vi "Main.vi"() -> ()   [LabVIEW 2021]
uses:
  <vilib>/Native 3D Graph/xcontrol/3DPC_SurfacePlot.xctl
  State.ctl
  CommCluster.ctl
  CommandCtrl.ctl
  DataCluster.ctl
  ToViewData.ctl
  ToViewCMD.ctl
panel:
  out "3D Graph":refnum<class "Base Datatype.lvclass">[](xcontrol)
  out "length":i32
  out "Stoping":bool
  in  "remote port or service name 2":u16=2137
  in  "address":string="192.168.0.1"
  in  "stop":bool
  in  "Str To Send":string
  out "ReceivedData":string
  in  "Send":bool
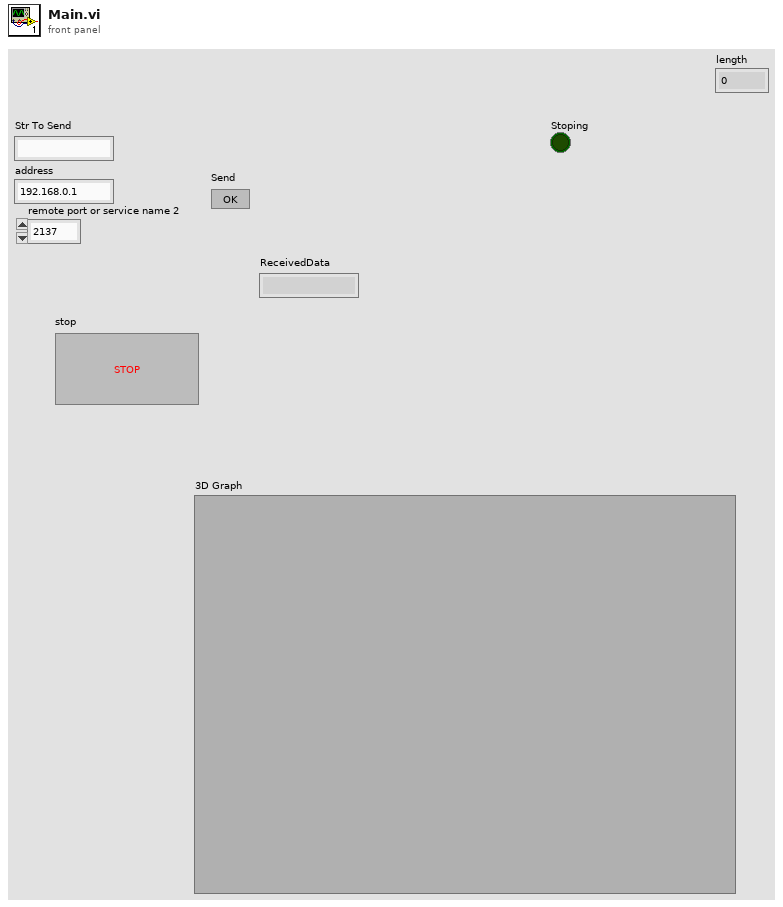
[diagram p1: front panel]
types:
  T1 = typedef "ToViewData.ctl" = cluster{"RecivedStr":string, "Enum":T2}
  T2 = typedef "ToViewCMD.ctl" = enum16{"Exit", "Init", "Update View"}
  T3 = typedef "DataCluster.ctl" = cluster{"connection ID":refnum<k5>, "Str to Send":string, "Received str":string}
  T4 = typedef "CommCluster.ctl" = cluster{"Command":T5, "Data":T3}
  T5 = typedef "CommandCtrl.ctl" = enum16{"Exit", "Init", "Receive TCP", "Send TCP"}
  T6 = typedef "State.ctl" = enum16{"Init", "Idle", "TCP_Read", "TCP_Write", "Exit"}
  T7 = enum16{"Standard", "Buffered", "CRLF", "Immediate"}
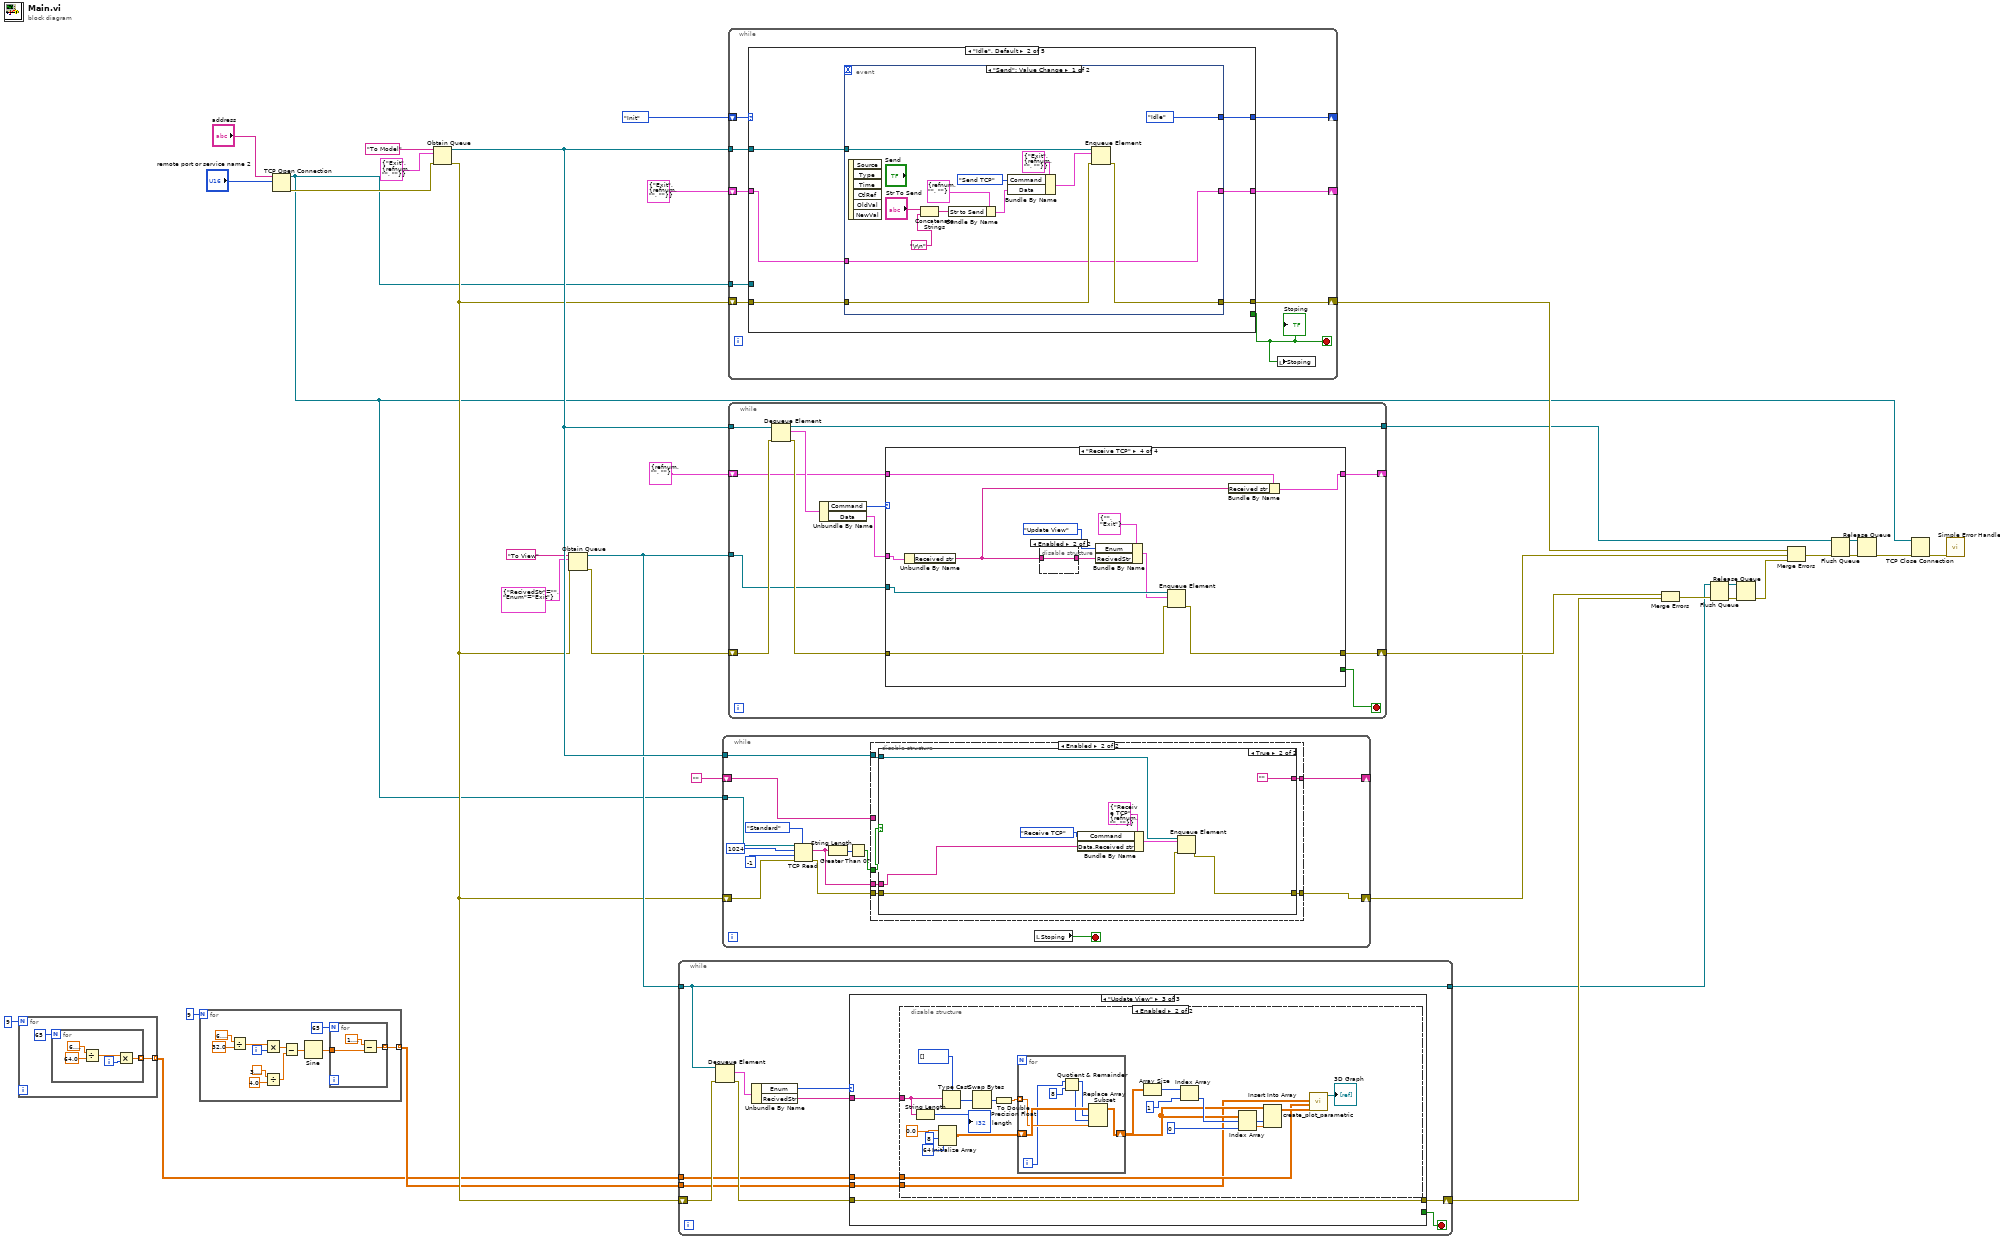
[diagram p0: block diagram]
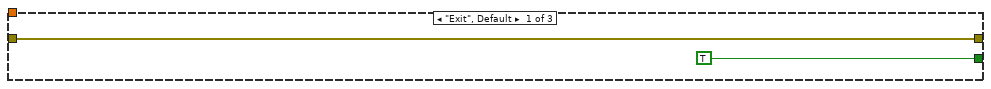
[diagram p2: hidden frame]
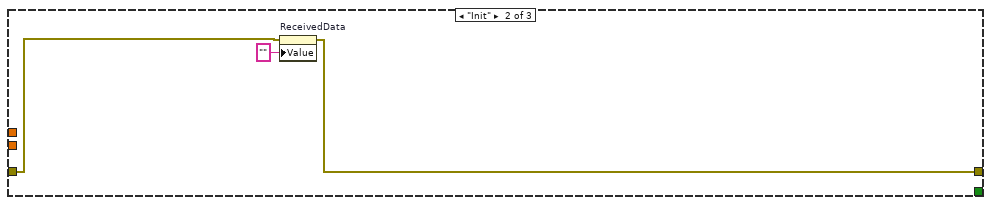
[diagram p3: hidden frame]
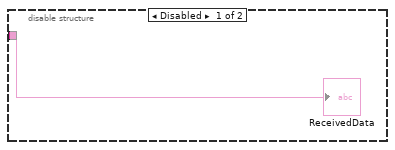
[diagram p4: hidden frame]
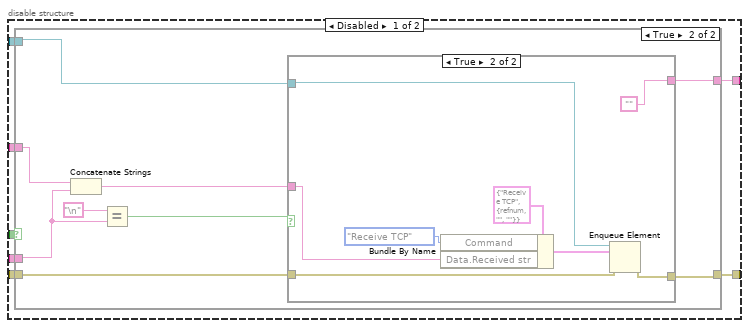
[diagram p5: hidden frame]
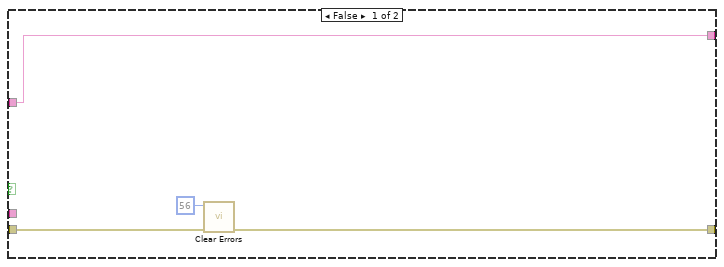
[diagram p6: hidden frame]
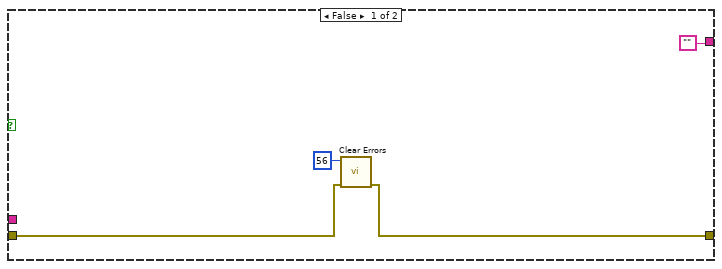
[diagram p8: hidden frame]
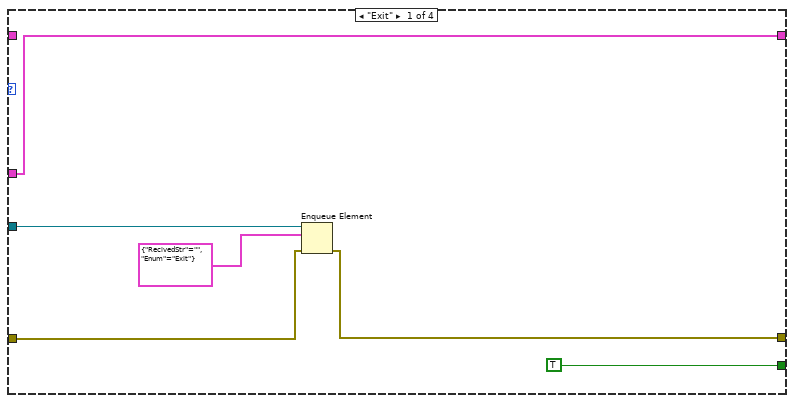
[diagram p9: hidden frame]
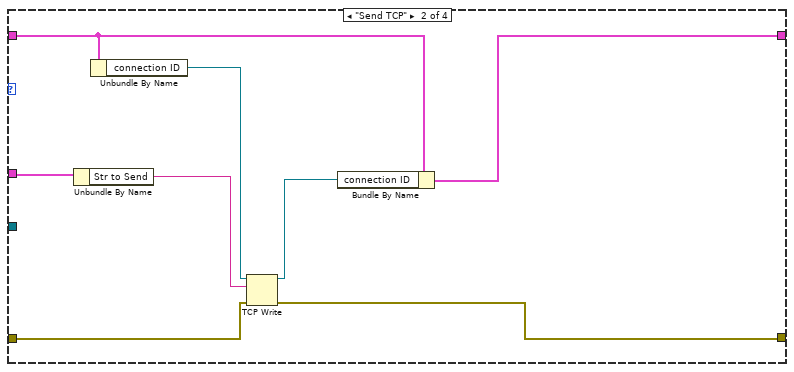
[diagram p10: hidden frame]
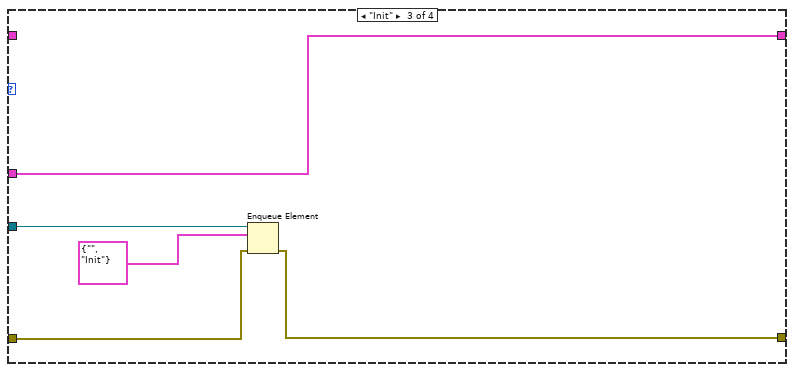
[diagram p11: hidden frame]
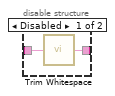
[diagram p12: hidden frame]
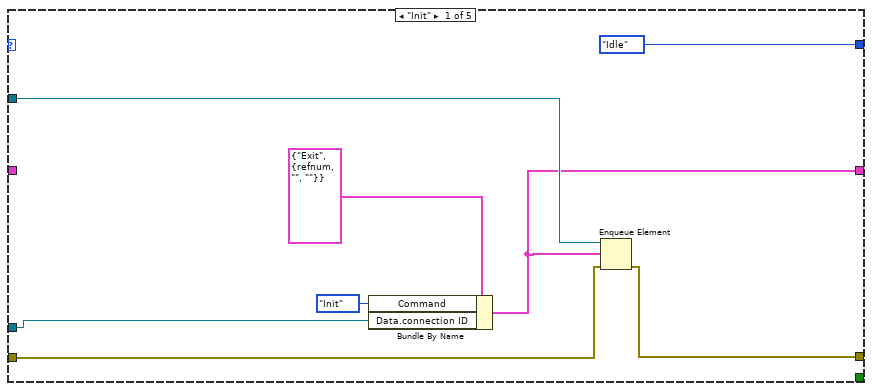
[diagram p13: hidden frame]
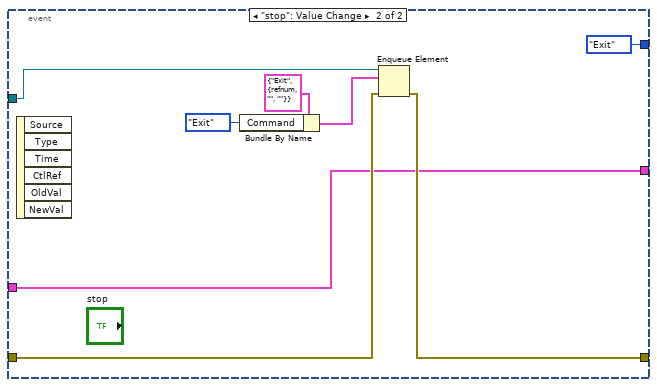
[diagram p14: hidden frame]
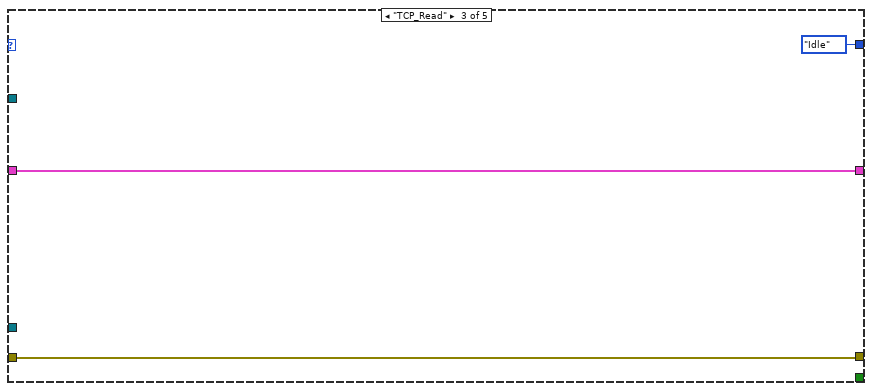
[diagram p15: hidden frame]
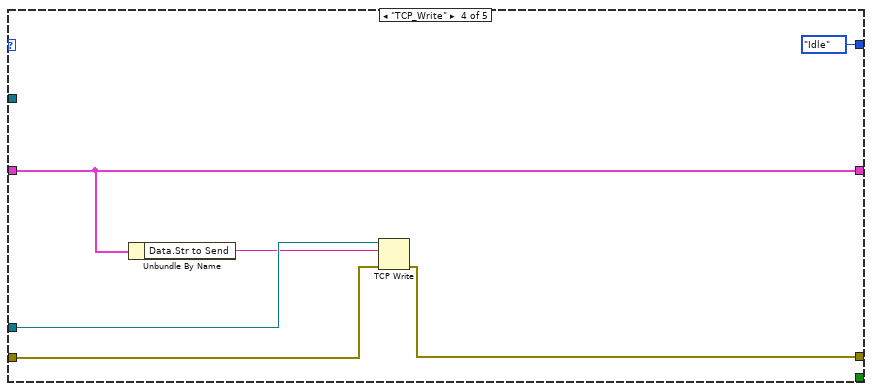
[diagram p16: hidden frame]
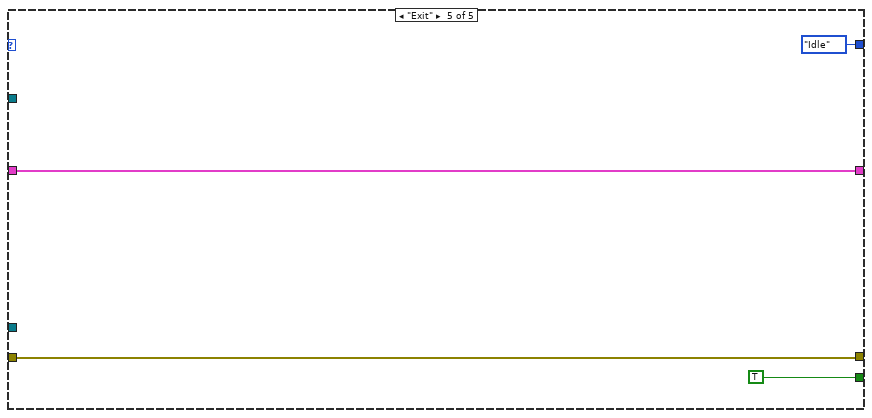
[diagram p17: hidden frame]
diagram:
  n1 = for {
    N: 9 -> [_]
    tunnel: [w36] -> w1 mode=indexing
    n2 = for {
      N: 65 -> [_]
      tunnel: [w39] -> w36 mode=indexing
      i -> [w40]
      n3 = Divide(x=6.283185307179586, y=64.0) -> (x/y=w41:dbl)
      n4 = Multiply(x=w41, y=w40) -> (x*y=w39:dbl)
    }
  }
  n5 = for {
    N: 9 -> [_]
    tunnel: [w44] -> w2 mode=indexing
    i -> [w52]
    n6 = Divide(x=6.283185307179586, y=32.0) -> (x/y=w53:dbl)
    n7 = Multiply(x=w53, y=w52) -> (x*y=w49:dbl)
    n8 = Divide(x=3.141592653589793, y=4.0) -> (x/y=w46:dbl)
    n9 = Subtract(x=w49, y=w46) -> (x-y=w50:dbl)
    n10 = Sine(x=w50) -> (sin(x)=w45:dbl)
    n11 = for {
      N: 65 -> [_]
      tunnel: w45 -> [w56]
      tunnel: [w55] -> w44 mode=indexing
      n12 = Subtract(x=1.5707963267948966, y=w56) -> (x-y=w55:dbl)
    }
  }
  n13 = TCP Open Connection(address="address", remote port or service name="remote port or service name 2") -> (connection ID=w6:refnum<k5>, error out=w28:errorcluster)  [unwired: 3 in]
  n14 = Obtain Queue(name (unnamed)="To Model", element data type=T4 {"Command"=enum."Exit", "Data"={"connection ID"=refnum, "Str to Send"="", "Received str"=""}}, error in (no error)=w28) -> (queue out=w27:refnum<queue>, error out=w22:errorcluster)  [unwired: 2 in, 1 out]
  n15 = Obtain Queue(name (unnamed)="To View", element data type=T1 {"RecivedStr"="", "Enum"=enum."Exit"}, error in (no error)=w22) -> (queue out=w23:refnum<queue>, error out=w25:errorcluster)  [unwired: 2 in, 1 out]
  n16 = while {
    shift-right: [w63] -> w21
    shift-left: w22 -> [w67]
    tunnel: w23 -> [w60]
    tunnel: [w60] -> w18
    tunnel: w2 -> [w59]
    tunnel: w1 -> [w58]
    stop <- w62 stop-if-true
    n17 = Dequeue Element(queue=w60, error in (no error)=w67) -> (element=w66:T1, error out=w64:errorcluster)  [unwired: 1 in, 2 out]
    n18 = Unbundle By Name(w66) -> ("Enum"=w65:T2, "RecivedStr"=w61:string)
    n19 = case shown="\"Update View\"" w65 {
      tunnel: w64 -> [w68 w71 w76]
      tunnel: [w68 w70 w76] -> w63
      tunnel: [TRUE _ _] -> w62
      tunnel: w61 -> [_ _ w75]
      tunnel: w59 -> [_ _ w74]
      tunnel: w58 -> [_ _ w73]
      frame "Exit", Default {
      }
      frame "Init" {
        n20 = property on="ReceivedData" class="Str"(error in=w71, "Value"="" ("ReceivedData")) -> (error out=w70:errorcluster)  [unwired: 1 in, 1 out]
      }
      frame "Update View" {
        n21 = disable-structure shown="Enabled" {
          disable-tunnel: w75 -> [w77 w90]
          disable-tunnel: w74 -> [_ w78]
          disable-tunnel: w73 -> [_ w79]
          frame Disabled {
            "ReceivedData" <- w77
          }
          frame Enabled {
            n22 = String Length(string=w90) -> (length=→"length":i32)
            n23 = Initialize Array(0.0 ("element"), 8 ("dimension size"), 64 ("dimension size")) -> (w91:dbl[][])
            n24 = Type Cast(type=u16[] [], x=w90) -> (*(type *) &x=w96:u16[])
            n25 = Swap Bytes(anything=w96) -> (byte swapped=w88:u16[])
            n26 = To Double Precision Float(number=w88) -> (double precision float=w95:dbl[])
            n27 = for {
              tunnel: w95 -> [w100] mode=indexing
              shift-right: [w102] -> w84
              shift-left: w91 -> [w104]
              i -> [w98]
              n28 = Quotient & Remainder(x=w98, y=8 ("x")) -> (x-y*floor(x/y)=w103:i32, floor(x/y)=w101:i32)
              n29 = Replace Array Subset(array=w104, new element=w100, index (row)=w103, index (col)=w101) -> (w102:dbl[][])
            }
            n30 = Array Size(array=w84) -> (size(s)=w87:i32[])
            n31 = Index Array(array=w87, index=1) -> (element=w85:i32)
            n32 = Index Array(array=w84, index (col)=0 ("disabled index (col)")) -> (element=w82:dbl[])  [unwired: 1 in]
            n33 = Insert Into Array(array=w84, index (col)=w85, new element=w82) -> (w80:dbl[][])  [unwired: 1 in]
            n34 = call <vilib>:"create_plot_parametric.vi"("z matrix"=w80, "y matrix"=w79, "x matrix"=w78) -> ("plots out"=→"3D Graph":refnum<class "Base Datatype.lvclass">[])  [unwired: 2 in, 6 out]
          }
        }
      }
    }
  }
  n35 = while {
    shift-right: [w109] -> w13
    shift-left: w22 -> [w116]
    tunnel: w27 -> [w111]
    tunnel: w6 -> [w117]
    shift-right: [w106] -> _
    shift-left: "" -> [w107]
    stop <- w115 stop-if-true
    n36 = TCP Read(connection ID=w117, bytes to read=1024, error in (no error)=w116, 7:T7."Standard" ("mode (standard)"), 9:-1 ("timeout ms (25000)")) -> (data out=w114:string, error out=w110:errorcluster)  [unwired: 1 out]
    n37 = String Length(string=w114) -> (length=w113:i32)
    n38 = Greater Than 0?(x=w113) -> (x > 0?=w112:bool)
    n39 = disable-structure shown="Enabled" {
      disable-tunnel: w114 -> [w125 w153]
      disable-tunnel: w112 -> [w124 w151]
      disable-tunnel: w111 -> [w123 w154]
      disable-tunnel: w110 -> [w122 w152]
      disable-tunnel: [w121 w150] -> w109
      disable-tunnel: w107 -> [w120 _]
      disable-tunnel: [w119 w149] -> w106
      frame Disabled {
        n40 = case shown="True" w124 {
          tunnel: w125 -> [_ w132]
          tunnel: w123 -> [_ w138]
          tunnel: w122 -> [w129 w137]
          tunnel: [w127 w136] -> w121
          tunnel: w120 -> [w128 w133]
          tunnel: [w128 w130] -> w119
          frame False {
            n41 = call <vilib>:"Clear Errors.vi"("error in (no error)"=w129, "specific error code to clear (0: all)"=56) -> ("error out"=w127:errorcluster)  [unwired: 4 in, 1 out]
          }
          frame True {
            n42 = Concatenate Strings(w133, w132) -> (w131:string)
            n43 = Equal?(x="\n", y=w132) -> (x = y?=w134:bool)
            n44 = case shown="True" w134 {
              tunnel: w138 -> [_ w146]
              tunnel: w137 -> [w139 w144]
              tunnel: [w139 w143] -> w136
              tunnel: w131 -> [w140 w142]
              tunnel: [w140 ""] -> w130
              frame False {
              }
              frame True {
                n45 = Bundle By Name(cluster=T4 {"Command"=enum."Receive TCP", "Data"={"connection ID"=refnum, "Str to Send"="", "Received str"=""}} ("element"), "Command"=CommandCtrl."Receive TCP", "Data.Received str"=w142) -> (w145:T4)
                n46 = Enqueue Element(queue=w146, element=w145, error in (no error)=w144) -> (error out=w143:errorcluster)  [unwired: 1 in, 2 out]
              }
            }
          }
        }
      }
      frame Enabled {
        n47 = case shown="True" w151 {
          tunnel: w154 -> [_ w160]
          tunnel: w153 -> [_ w163]
          tunnel: w152 -> [w157 w162]
          tunnel: [w156 w161] -> w150
          tunnel: ["" ""] -> w149
          frame False {
            n48 = call <vilib>:"Clear Errors.vi"("error in (no error)"=w157, "specific error code to clear (0: all)"=56) -> ("error out"=w156:errorcluster)  [unwired: 4 in, 1 out]
          }
          frame True {
            n49 = Bundle By Name(cluster=T4 {"Command"=enum."Receive TCP", "Data"={"connection ID"=refnum, "Str to Send"="", "Received str"=""}} ("element"), "Command"=CommandCtrl."Receive TCP", "Data.Received str"=w163) -> (w164:T4)
            n50 = Enqueue Element(queue=w160, element=w164, error in (no error)=w162) -> (error out=w161:errorcluster)  [unwired: 1 in, 2 out]
          }
        }
      }
    }
    n51 = local read "Stoping"() -> (w115:bool)
  }
  n52 = while {
    shift-right: [w170] -> _
    shift-left: State."Init" -> [w175]
    shift-right: [w174] -> w14
    shift-left: w22 -> [w173]
    shift-right: [w171] -> _
    shift-left: T4 {"Command"=enum."Exit", "Data"={"connection ID"=refnum, "Str to Send"="", "Received str"=""}} -> [w172]
    tunnel: w6 -> [w168]
    tunnel: w27 -> [w169]
    stop <- w167 stop-if-true
    n53 = case shown="\"Idle\", Default" w175 {
      tunnel: [_ _ _ _ TRUE] -> w167
      tunnel: [w178 w188 w213 w216 w222] -> w174
      tunnel: w173 -> [w183 w189 w213 w217 w222]
      tunnel: w172 -> [_ w186 w212 w215 w221]
      tunnel: [w177 w185 w212 w215 w221] -> w171
      tunnel: [State."Idle" w184 State."Idle" State."Idle" State."Idle"] -> w170
      tunnel: w169 -> [w180 w187 _ _ _]
      tunnel: w168 -> [w176 _ _ w218 _]
      frame "Init" {
        n54 = Bundle By Name(cluster=T4 {"Command"=enum."Exit", "Data"={"connection ID"=refnum, "Str to Send"="", "Received str"=""}}, "Command"=CommandCtrl."Init", "Data.connection ID"=w176) -> (w177:T4)
        n55 = Enqueue Element(queue=w180, element=w177, error in (no error)=w183) -> (error out=w178:errorcluster)  [unwired: 1 in, 2 out]
      }
      frame "Idle", Default {
        n56 = event shown="[0] \"Send\": Value Change" {
          selector: _ -> [_ _]
          dyn-events: _ -> [_ _]
          timeout: _ -> [_ _]
          tunnel: w189 -> [w193 w206]
          tunnel: [w192 w205] -> w188
          tunnel: w187 -> [w202 w207]
          tunnel: w186 -> [w191 w204]
          tunnel: [w191 w204] -> w185
          tunnel: [State."Idle" State."Exit"] -> w184
          event "Send": Value Change {
            n57 = event-data() -> ()  [unwired: 1 in, 6 out]
            n58 = Concatenate Strings("Str To Send", "\r\n") -> (w195:string)
            n59 = Bundle By Name(cluster=T3 {"connection ID"=refnum, "Str to Send"="", "Received str"=""} ("Data"), "Str to Send"=w195) -> (w198:T3)
            n60 = Bundle By Name(cluster=T4 {"Command"=enum."Exit", "Data"={"connection ID"=refnum, "Str to Send"="", "Received str"=""}}, "Command"=CommandCtrl."Send TCP", "Data"=w198) -> (w201:T4)
            n61 = Enqueue Element(queue=w202, element=w201, error in (no error)=w193) -> (error out=w192:errorcluster)  [unwired: 1 in, 2 out]
          }
          event "stop": Value Change {
            n62 = event-data() -> ()  [unwired: 1 in, 6 out]
            n63 = Bundle By Name(cluster=T4 {"Command"=enum."Exit", "Data"={"connection ID"=refnum, "Str to Send"="", "Received str"=""}}, "Command"=CommandCtrl."Exit") -> (w210:T4)
            n64 = Enqueue Element(queue=w207, element=w210, error in (no error)=w206) -> (error out=w205:errorcluster)  [unwired: 1 in, 2 out]
          }
        }
      }
      frame "TCP_Read" {
      }
      frame "TCP_Write" {
        n65 = Unbundle By Name(w215) -> ("Data.Str to Send"=w214:string)
        n66 = TCP Write(connection ID=w218, data in=w214, error in (no error)=w217) -> (error out=w216:errorcluster)  [unwired: 1 in, 2 out]
      }
      frame "Exit" {
      }
    }
    "Stoping" <- w167
    n67 = local write "Stoping"(w167) -> ()
  }
  n68 = while {
    shift-right: [w227] -> _
    shift-left: T3 {"connection ID"=refnum, "Str to Send"="", "Received str"=""} ("Data") -> [w228]
    shift-right: [w226] -> w20
    shift-left: w25 -> [w234]
    tunnel: w23 -> [w225]
    tunnel: w27 -> [w235]
    tunnel: [w224] -> w10
    stop <- w230 stop-if-true
    n69 = Dequeue Element(queue=w235, error in (no error)=w234) -> (queue out=w224:refnum<queue>, element=w232:T4, error out=w233:errorcluster)  [unwired: 1 in, 1 out]
    n70 = Unbundle By Name(w232) -> ("Command"=w231:T5, "Data"=w229:T3)
    n71 = case shown="\"Receive TCP\"" w231 {
      tunnel: w233 -> [w238 w249 w252 w261]
      tunnel: [TRUE _ _ _] -> w230
      tunnel: w229 -> [w240 w247 w254 w265]
      tunnel: w228 -> [_ w242 _ w264]
      tunnel: [w240 w245 w254 w263] -> w227
      tunnel: [w237 w244 w251 w260] -> w226
      tunnel: w225 -> [w239 _ w253 w262]
      frame "Exit" {
        n72 = Enqueue Element(queue=w239, element=T1 {"RecivedStr"="", "Enum"=enum."Exit"}, error in (no error)=w238) -> (error out=w237:errorcluster)  [unwired: 1 in, 2 out]
      }
      frame "Send TCP" {
        n73 = Unbundle By Name(w247) -> ("Str to Send"=w248:string)
        n74 = Unbundle By Name(w242) -> ("connection ID"=w243:refnum<k5>)
        n75 = TCP Write(connection ID=w243, data in=w248, error in (no error)=w249) -> (connection ID out=w246:refnum<k5>, error out=w244:errorcluster)  [unwired: 1 in, 1 out]
        n76 = Bundle By Name(cluster=w242, "connection ID"=w246) -> (w245:T3)
      }
      frame "Init" {
        n77 = Enqueue Element(queue=w253, element=T1 {"RecivedStr"="", "Enum"=enum."Init"}, error in (no error)=w252) -> (error out=w251:errorcluster)  [unwired: 1 in, 2 out]
      }
      frame "Receive TCP" {
        n78 = Unbundle By Name(w265) -> ("Received str"=w259:string)
        n79 = disable-structure shown="Enabled" {
          disable-tunnel: w259 -> [w267 w268]
          disable-tunnel: [w266 w268] -> w255
          frame Disabled {
            n80 = call <vilib>:"Trim Whitespace.vi"("string"=w267) -> ("trimmed string"=w266:string)  [unwired: 1 in]
          }
          frame Enabled {
          }
        }
        n81 = Bundle By Name(cluster=T1 {"RecivedStr"="", "Enum"=enum."Exit"}, "Enum"=ToViewCMD."Update View", "RecivedStr"=w255) -> (w256:T1)
        n82 = Enqueue Element(queue=w262, element=w256, error in (no error)=w261) -> (error out=w260:errorcluster)  [unwired: 1 in, 2 out]
        n83 = Bundle By Name(cluster=w264, "Received str"=w259) -> (w263:T3)
      }
    }
  }
  n84 = Merge Errors(w20, w21) -> (w19:errorcluster)
  n85 = Flush Queue(queue=w18, error in (no error)=w19) -> (queue out=w16:refnum<queue>, error out=w17:errorcluster)  [unwired: 1 out]
  n86 = Release Queue(queue=w16, error in (no error)=w17) -> (error out=w15:errorcluster)  [unwired: 1 in, 2 out]
  n87 = Merge Errors(w14, w13, w15) -> (w11:errorcluster)
  n88 = Flush Queue(queue=w10, error in (no error)=w11) -> (queue out=w9:refnum<queue>, error out=w12:errorcluster)  [unwired: 1 out]
  n89 = Release Queue(queue=w9, error in (no error)=w12) -> (error out=w7:errorcluster)  [unwired: 1 in, 2 out]
  n90 = TCP Close Connection(connection ID=w6, error in (no error)=w7) -> (error out=w8:errorcluster)  [unwired: 1 in, 1 out]
  n91 = call <vilib>:"Simple Error Handler.vi"("error in (no error)"=w8) -> ()  [unwired: 4 in, 5 out]
